vi "Get Active List - By Core Number.vi"(7 "Parameters Array (in)":T1[](array[typedef])) -> (8 "Active Core Numbers":i32[](array[numeric]))   [LabVIEW 2017] (continued)
Number"=0, "Channel Number"=8, "Channel Name"="RDC13_NWS_RX", "Channel Speed"=100, "Label Decimal"=6, "Label Name"="Label_6", "Min Rate (mS)"=40, "Max Rate (mS)"=60, "SDI"=0, "SSM"=0, "Create SDI"=FALSE, "Create SSM"=FALSE, "Create Parity"=FALSE, "Parameter Name"="left_wheel_speed", "Start Bit"=16, "Number of Bits"=13, "Scale"="0.125", "Offset"="0", "Signed"=TRUE, "Unit"="knots", "Encoding"=enum."BNR", "Default Value"="0"}, {"Core Number"=0, "Channel Number"=8, "Channel Name"="RDC13_NWS_RX", "Channel Speed"=100, "Label Decimal"=6, "Label Name"="Label_6", "Min Rate (mS)"=40, "Max Rate (mS)"=60, "SDI"=0, "SSM"=0, "Create SDI"=FALSE, "Create SSM"=FALSE, "Create Parity"=FALSE, "Parameter Name"="sdi", "Start Bit"=8, "Number of Bits"=2, "Scale"="1", "Offset"="0", "Signed"=FALSE, "Unit"="", "Encoding"=enum."BNR", "Default Value"="0"}, {"Core Number"=0, "Channel Number"=8, "Channel Name"="RDC13_NWS_RX", "Channel Speed"=100, "Label Decimal"=7, "Label Name"="Label_7", "Min Rate (mS)"=40, "Max Rate (mS)"=60, "SDI"=0, "SSM"=0, "Create SDI"=FALSE, "Create SSM"=FALSE, "Create Parity"=FALSE, "Parameter Name"="right_wheel_speed", "Start Bit"=16, "Number of Bits"=13, "Scale"="0.125", "Offset"="0", "Signed"=TRUE, "Unit"="knots", "Encoding"=enum."BNR", "Default Value"="0"}, {"Core Number"=0, "Channel Number"=8, "Channel Name"="RDC13_NWS_RX", "Channel Speed"=100, "Label Decimal"=7, "Label Name"="Label_7", "Min Rate (mS)"=40, "Max Rate (mS)"=60, "SDI"=0, "SSM"=0, "Create SDI"=FALSE, "Create SSM"=FALSE, "Create Parity"=FALSE, "Parameter Name"="sdi", "Start Bit"=8, "Number of Bits"=2, "Scale"="1", "Offset"="0", "Signed"=FALSE, "Unit"="", "Encoding"=enum."BNR", "Default Value"="0"}, {"Core Number"=0, "Channel Number"=8, "Channel Name"="RDC13_NWS_RX", "Channel Speed"=100, "Label Decimal"=17, "Label Name"="Label_21", "Min Rate (mS)"=16, "Max Rate (mS)"=24, "SDI"=0, "SSM"=0, "Create SDI"=FALSE, "Create SSM"=FALSE, "Create Parity"=FALSE, "Parameter Name"="gear_down_select", "Start Bit"=26, "Number of Bits"=1, "Scale"="0", "Offset"="0", "Signed"=FALSE, "Unit"="", "Encoding"=enum."Discrete", "Default Value"="0"}, {"Core Number"=0, "Channel Number"=8, "Channel Name"="RDC13_NWS_RX", "Channel Speed"=100, "Label Decimal"=17, "Label Name"="Label_21", "Min Rate (mS)"=16, "Max Rate (mS)"=24, "SDI"=0, "SSM"=0, "Create SDI"=FALSE, "Create SSM"=FALSE, "Create Parity"=FALSE, "Parameter Name"="gear_in_transit_state", "Start Bit"=24, "Number of Bits"=1, "Scale"="0", "Offset"="0", "Signed"=FALSE, "Unit"="", "Encoding"=enum."Discrete", "Default Value"="0"}, {"Core Number"=0, "Channel Number"=8, "Channel Name"="RDC13_NWS_RX", "Channel Speed"=100, "Label Decimal"=17, "Label Name"="Label_21", "Min Rate (mS)"=16, "Max Rate (mS)"=24, "SDI"=0, "SSM"=0, "Create SDI"=FALSE, "Create SSM"=FALSE, "Create Parity"=FALSE, "Parameter Name"="gear_up_select", "Start Bit"=27, "Number of Bits"=1, "Scale"="0", "Offset"="0", "Signed"=FALSE, "Unit"="", "Encoding"=enum."Discrete", "Default Value"="0"}, {"Core Number"=0, "Channel Number"=8, "Channel Name"="RDC13_NWS_RX", "Channel Speed"=100, "Label Decimal"=17, "Label Name"="Label_21", "Min Rate (mS)"=16, "Max Rate (mS)"=24, "SDI"=0, "SSM"=0, "Create SDI"=FALSE, "Create SSM"=FALSE, "Create Parity"=FALSE, "Parameter Name"="lh_mlg_gear_downlock_state", "Start Bit"=18, "Number of Bits"=1, "Scale"="0", "Offset"="0", "Signed"=FALSE, "Unit"="", "Encoding"=enum."Discrete", "Default Value"="0"}, {"Core Number"=0, "Channel Number"=8, "Channel Name"="RDC13_NWS_RX", "Channel Speed"=100, "Label Decimal"=17, "Label Name"="Label_21", "Min Rate (mS)"=16, "Max Rate (mS)"=24, "SDI"=0, "SSM"=0, "Create SDI"=FALSE, "Create SSM"=FALSE, "Create Parity"=FALSE, "Parameter Name"="lh_mlg_gear_downlock_valid", "Start Bit"=19, "Number of Bits"=1, "Scale"="0", "Offset"="0", "Signed"=FALSE, "Unit"="", "Encoding"=enum."Discrete", "Default Value"="0"}, {"Core Number"=0, "Channel Number"=8, "Channel Name"="RDC13_NWS_RX", "Channel Speed"=100, "Label Decimal"=17, "Label Name"="Label_21", "Min Rate (mS)"=16, "Max Rate (mS)"=24, "SDI"=0, "SSM"=0, "Create SDI"=FALSE, "Create SSM"=FALSE, "Create Parity"=FALSE, "Parameter Name"="lh_mlg_gear_uplock_state", "Start Bit"=10, "Number of Bits"=1, "Scale"="0", "Offset"="0", "Signed"=FALSE, "Unit"="", "Encoding"=enum."Discrete", "Default Value"="0"}, {"Core Number"=0, "Channel Number"=8, "Channel Name"="RDC13_NWS_RX", "Channel Speed"=100, "Label Decimal"=17, "Label Name"="Label_21", "Min Rate (mS)"=16, "Max Rate (mS)"=24, "SDI"=0, "SSM"=0, "Create SDI"=FALSE, "Create SSM"=FALSE, "Create Parity"=FALSE, "Parameter Name"="lh_mlg_gear_uplock_valid", "Start Bit"=11, "Number of Bits"=1, "Scale"="0", "Offset"="0", "Signed"=FALSE, "Unit"="", "Encoding"=enum."Discrete", "Default Value"="0"}, {"Core Number"=0, "Channel Number"=8, "Channel Name"="RDC13_NWS_RX", "Channel Speed"=100, "Label Decimal"=17, "Label Name"="Label_21", "Min Rate (mS)"=16, "Max Rate (mS)"=24, "SDI"=0, "SSM"=0, "Create SDI"=FALSE, "Create SSM"=FALSE, "Create Parity"=FALSE, "Parameter Name"="maint_mode_mlg_extend_selected", "Start Bit"=28, "Number of Bits"=1, "Scale"="0", "Offset"="0", "Signed"=FALSE, "Unit"="", "Encoding"=enum."Discrete", "Default Value"="0"}, {"Core Number"=0, "Channel Number"=8, "Channel Name"="RDC13_NWS_RX", "Channel Speed"=100, "Label Decimal"=17, "Label Name"="Label_21", "Min Rate (mS)"=16, "Max Rate (mS)"=24, "SDI"=0, "SSM"=0, "Create SDI"=FALSE, "Create SSM"=FALSE, "Create Parity"=FALSE, "Parameter Name"="maint_mode_mlg_retract_selected", "Start Bit"=17, "Number of Bits"=1, "Scale"="0", "Offset"="0", "Signed"=FALSE, "Unit"="", "Encoding"=enum."Discrete", "Default Value"="0"}, {"Core Number"=0, "Channel Number"=8, "Channel Name"="RDC13_NWS_RX", "Channel Speed"=100, "Label Decimal"=17, "Label Name"="Label_21", "Min Rate (mS)"=16, "Max Rate (mS)"=24, "SDI"=0, "SSM"=0, "Create SDI"=FALSE, "Create SSM"=FALSE, "Create Parity"=FALSE, "Parameter Name"="nlg_gear_downlock_state", "Start Bit"=22, "Number of Bits"=1, "Scale"="0", "Offset"="0", "Signed"=FALSE, "Unit"="", "Encoding"=enum."Discrete", "Default Value"="0"}, {"Core Number"=0, "Channel Number"=8, "Channel Name"="RDC13_NWS_RX", "Channel Speed"=100, "Label Decimal"=17, "Label Name"="Label_21", "Min Rate (mS)"=16, "Max Rate (mS)"=24, "SDI"=0, "SSM"=0, "Create SDI"=FALSE, "Create SSM"=FALSE, "Create Parity"=FALSE, "Parameter Name"="nlg_gear_downlock_valid", "Start Bit"=23, "Number of Bits"=1, "Scale"="0", "Offset"="0", "Signed"=FALSE, "Unit"="", "Encoding"=enum."Discrete", "Default Value"="0"}, {"Core Number"=0, "Channel Number"=8, "Channel Name"="RDC13_NWS_RX", "Channel Speed"=100, "Label Decimal"=17, "Label Name"="Label_21", "Min Rate (mS)"=16, "Max Rate (mS)"=24, "SDI"=0, "SSM"=0, "Create SDI"=FALSE, "Create SSM"=FALSE, "Create Parity"=FALSE, "Parameter Name"="nlg_gear_uplock_state", "Start Bit"=14, "Number of Bits"=1, "Scale"="0", "Offset"="0", "Signed"=FALSE, "Unit"="", "Encoding"=enum."Discrete", "Default Value"="0"}, {"Core Number"=0, "Channel Number"=8, "Channel Name"="RDC13_NWS_RX", "Channel Speed"=100, "Label Decimal"=17, "Label Name"="Label_21", "Min Rate (mS)"=16, "Max Rate (mS)"=24, "SDI"=0, "SSM"=0, "Create SDI"=FALSE, "Create SSM"=FALSE, "Create Parity"=FALSE, "Parameter Name"="nlg_gear_uplock_valid", "Start Bit"=15, "Number of Bits"=1, "Scale"="0", "Offset"="0", "Signed"=FALSE, "Unit"="", "Encoding"=enum."Discrete", "Default Value"="0"}, {"Core Number"=0, "Channel Number"=8, "Channel Name"="RDC13_NWS_RX", "Channel Speed"=100, "Label Decimal"=17, "Label Name"="Label_21", "Min Rate (mS)"=16, "Max Rate (mS)"=24, "SDI"=0, "SSM"=0, "Create SDI"=FALSE, "Create SSM"=FALSE, "Create Parity"=FALSE, "Parameter Name"="nose_wheel_centered", "Start Bit"=16, "Number of Bits"=1, "Scale"="0", "Offset"="0", "Signed"=FALSE, "Unit"="", "Encoding"=enum."Discrete", "Default Value"="0"}, {"Core Number"=0, "Channel Number"=8, "Channel Name"="RDC13_NWS_RX", "Channel Speed"=100, "Label Decimal"=17, "Label Name"="Label_21", "Min Rate (mS)"=16, "Max Rate (mS)"=24, "SDI"=0, "SSM"=0, "Create SDI"=FALSE, "Create SSM"=FALSE, "Create Parity"=FALSE, "Parameter Name"="rh_mlg_gear_downlock_state", "Start Bit"=20, "Number of Bits"=1, "Scale"="0", "Offset"="0", "Signed"=FALSE, "Unit"="", "Encoding"=enum."Discrete", "Default Value"="0"}, {"Core Number"=0, "Channel Number"=8, "Channel Name"="RDC13_NWS_RX", "Channel Speed"=100, "Label Decimal"=17, "Label Name"="Label_21", "Min Rate (mS)"=16, "Max Rate (mS)"=24, "SDI"=0, "SSM"=0, "Create SDI"=FALSE, "Create SSM"=FALSE, "Create Parity"=FALSE, "Parameter Name"="rh_mlg_gear_downlock_valid", "Start Bit"=21, "Number of Bits"=1, "Scale"="0", "Offset"="0", "Signed"=FALSE, "Unit"="", "Encoding"=enum."Discrete", "Default Value"="0"}, {"Core Number"=0, "Channel Number"=8, "Channel Name"="RDC13_NWS_RX", "Channel Speed"=100, "Label Decimal"=17, "Label Name"="Label_21", "Min Rate (mS)"=16, "Max Rate (mS)"=24, "SDI"=0, "SSM"=0, "Create SDI"=FALSE, "Create SSM"=FALSE, "Create Parity"=FALSE, "Parameter Name"="rh_mlg_gear_uplock_state", "Start Bit"=12, "Number of Bits"=1, "Scale"="0", "Offset"="0", "Signed"=FALSE, "Unit"="", "Encoding"=enum."Discrete", "Default Value"="0"}, {"Core Number"=0, "Channel Number"=8, "Channel Name"="RDC13_NWS_RX", "Channel Speed"=100, "Label Decimal"=17, "Label Name"="Label_21", "Min Rate (mS)"=16, "Max Rate (mS)"=24, "SDI"=0, "SSM"=0, "Create SDI"=FALSE, "Create SSM"=FALSE, "Create Parity"=FALSE, "Parameter Name"="rh_mlg_gear_uplock_valid", "Start Bit"=13, "Number of Bits"=1, "Scale"="0", "Offset"="0", "Signed"=FALSE, "Unit"="", "Encoding"=enum."Discrete", "Default Value"="0"}, {"Core Number"=0, "Channel Number"=8, "Channel Name"="RDC13_NWS_RX", "Channel Speed"=100, "Label Decimal"=17, "Label Name"="Label_21", "Min Rate (mS)"=16, "Max Rate (mS)"=24, "SDI"=0, "SSM"=0, "Create SDI"=FALSE, "Create SSM"=FALSE, "Create Parity"=FALSE, "Parameter Name"="sdi", "Start Bit"=8, "Number of Bits"=2, "Scale"="1", "Offset"="0", "Signed"=FALSE, "Unit"="", "Encoding"=enum."BNR", "Default Value"="0"}, {"Core Number"=0, "Channel Number"=8, "Channel Name"="RDC13_NWS_RX", "Channel Speed"=100, "Label Decimal"=18, "Label Name"="Label_22", "Min Rate (mS)"=16, "Max Rate (mS)"=24, "SDI"=0, "SSM"=0, "Create SDI"=FALSE, "Create SSM"=FALSE, "Create Parity"=FALSE, "Parameter Name"="all_gear_not_uplocked_state", "Start Bit"=22, "Number of Bits"=1, "Scale"="0", "Offset"="0", "Signed"=FALSE, "Unit"="", "Encoding"=enum."Discrete", "Default Value"="0"}, {"Core Number"=0, "Channel Number"=8, "Channel Name"="RDC13_NWS_RX", "Channel Speed"=100, "Label Decimal"=18, "Label Name"="Label_22", "Min Rate (mS)"=16, "Max Rate (mS)"=24, "SDI"=0, "SSM"=0, "Create SDI"=FALSE, "Create SSM"=FALSE, "Create Parity"=FALSE, "Parameter Name"="all_gear_not_uplocked_valid", "Start Bit"=23, "Number of Bits"=1, "Scale"="0", "Offset"="0", "Signed"=FALSE, "Unit"="", "Encoding"=enum."Discrete", "Default Value"="0"}, {"Core Number"=0, "Channel Number"=8, "Channel Name"="RDC13_NWS_RX", "Channel Speed"=100, "Label Decimal"=18, "Label Name"="Label_22", "Min Rate (mS)"=16, "Max Rate (mS)"=24, "SDI"=0, "SSM"=0, "Create SDI"=FALSE, "Create SSM"=FALSE, "Create Parity"=FALSE, "Parameter Name"="comb_l_or_r_main_gear_downlocked_state", "Start Bit"=16, "Number of Bits"=1, "Scale"="0", "Offset"="0", "Signed"=FALSE, "Unit"="", "Encoding"=enum."Discrete", "Default Value"="0"}, {"Core Number"=0, "Channel Number"=8, "Channel Name"="RDC13_NWS_RX", "Channel Speed"=100, "Label Decimal"=18, "Label Name"="Label_22", "Min Rate (mS)"=16, "Max Rate (mS)"=24, "SDI"=0, "SSM"=0, "Create SDI"=FALSE, "Create SSM"=FALSE, "Create Parity"=FALSE, "Parameter Name"="comb_l_or_r_main_gear_downlocked_valid", "Start Bit"=17, "Number of Bits"=1, "Scale"="0", "Offset"="0", "Signed"=FALSE, "Unit"="", "Encoding"=enum."Discrete", "Default Value"="0"}, {"Core Number"=0, "Channel Number"=8, "Channel Name"="RDC13_NWS_RX", "Channel Speed"=100, "Label Decimal"=18, "Label Name"="Label_22", "Min Rate (mS)"=16, "Max Rate (mS)"=24, "SDI"=0, "SSM"=0, "Create SDI"=FALSE, "Create SSM"=FALSE, "Create Parity"=FALSE, "Parameter Name"="comb_lh_or_rh_mlg_not_wow", "Start Bit"=20, "Number of Bits"=1, "Scale"="0", "Offset"="0", "Signed"=FALSE, "Unit"="", "Encoding"=enum."Discrete", "Default Value"="0"}, {"Core Number"=0, "Channel Number"=8, "Channel Name"="RDC13_NWS_RX", "Channel Speed"=100, "Label Decimal"=18, "Label Name"="Label_22", "Min Rate (mS)"=16, "Max Rate (mS)"=24, "SDI"=0, "SSM"=0, "Create SDI"=FALSE, "Create SSM"=FALSE, "Create Parity"=FALSE, "Parameter Name"="comb_lh_or_rh_mlg_wow", "Start Bit"=18, "Number of Bits"=1, "Scale"="0", "Offset"="0", "Signed"=FALSE, "Unit"="", "Encoding"=enum."Discrete", "Default Value"="0"}, {"Core Number"=0, "Channel Number"=8, "Channel Name"="RDC13_NWS_RX", "Channel Speed"=100, "Label Decimal"=18, "Label Name"="Label_22", "Min Rate (mS)"=16, "Max Rate (mS)"=24, "SDI"=0, "SSM"=0, "Create SDI"=FALSE, "Create SSM"=FALSE, "Create Parity"=FALSE, "Parameter Name"="lh_mlg_wow_state", "Start Bit"=10, "Number of Bits"=1, "Scale"="0", "Offset"="0", "Signed"=FALSE, "Unit"="", "Encoding"=enum."Discrete", "Default Value"="0"}, {"Core Number"=0, "Channel Number"=8, "Channel Name"="RDC13_NWS_RX", "Channel Speed"=100, "Label Decimal"=18, "Label Name"="Label_22", "Min Rate (mS)"=16, "Max Rate (mS)"=24, "SDI"=0, "SSM"=0, "Create SDI"=FALSE, "Create SSM"=FALSE, "Create Parity"=FALSE, "Parameter Name"="lh_mlg_wow_valid", "Start Bit"=11, "Number of Bits"=1, "Scale"="0", "Offset"="0", "Signed"=FALSE, "Unit"="", "Encoding"=enum."Discrete", "Default Value"="0"}, {"Core Number"=0, "Channel Number"=8, "Channel Name"="RDC13_NWS_RX", "Channel Speed"=100, "Label Decimal"=18, "Label Name"="Label_22", "Min Rate (mS)"=16, "Max Rate (mS)"=24, "SDI"=0, "SSM"=0, "Create SDI"=FALSE, "Create SSM"=FALSE, "Create Parity"=FALSE, "Parameter Name"="lh_or_rh_mlg_not_wow_valid", "Start Bit"=21, "Number of Bits"=1, "Scale"="0", "Offset"="0", "Signed"=FALSE, "Unit"="", "Encoding"=enum."Discrete", "Default Value"="0"}, {"Core Number"=0, "Channel Number"=8, "Channel Name"="RDC13_NWS_RX", "Channel Speed"=100, "Label Decimal"=18, "Label Name"="Label_22", "Min Rate (mS)"=16, "Max Rate (mS)"=24, "SDI"=0, "SSM"=0, "Create SDI"=FALSE, "Create SSM"=FALSE, "Create Parity"=FALSE, "Parameter Name"="lh_or_rh_mlg_wow_valid", "Start Bit"=19, "Number of Bits"=1, "Scale"="0", "Offset"="0", "Signed"=FALSE, "Unit"="", "Encoding"=enum."Discrete", "Default Value"="0"}, {"Core Number"=0, "Channel Number"=8, "Channel Name"="RDC13_NWS_RX", "Channel Speed"=100, "Label Decimal"=18, "Label Name"="Label_22", "Min Rate (mS)"=16, "Max Rate (mS)"=24, "SDI"=0, "SSM"=0, "Create SDI"=FALSE, "Create SSM"=FALSE, "Create Parity"=FALSE, "Parameter Name"="maint_mode_nlg_extend_selected", "Start Bit"=25, "Number of Bits"=1, "Scale"="0", "Offset"="0", "Signed"=FALSE, "Unit"="", "Encoding"=enum."Discrete", "Default Value"="0"}, {"Core Number"=0, "Channel Number"=8, "Channel Name"="RDC13_NWS_RX", "Channel Speed"=100, "Label Decimal"=18, "Label Name"="Label_22", "Min Rate (mS)"=16, "Max Rate (mS)"=24, "SDI"=0, "SSM"=0, "Create SDI"=FALSE, "Create SSM"=FALSE, "Create Parity"=FALSE, "Parameter Name"="maint_mode_nlg_retract_selected", "Start Bit"=24, "Number of Bits"=1, "Scale"="0", "Offset"="0", "Signed"=FALSE, "Unit"="", "Encoding"=enum."Discrete", "Default Value"="0"}, {"Core Number"=0, "Channel Number"=8, "Channel Name"="RDC13_NWS_RX", "Channel Speed"=100, "Label Decimal"=18, "Label Name"="Label_22", "Min Rate (mS)"=16, "Max Rate (mS)"=24, "SDI"=0, "SSM"=0, "Create SDI"=FALSE, "Create SSM"=FALSE, "Create Parity"=FALSE, "Parameter Name"="maint_mode_selected", "Start Bit"=28, "Number of Bits"=1, "Scale"="0", "Offset"="0", "Signed"=FALSE, "Unit"="", "Encoding"=enum."Discrete", "Default Value"="0"}, {"Core Number"=0, "Channel Number"=8, "Channel Name"="RDC13_NWS_RX", "Channel Speed"=100, "Label Decimal"=18, "Label Name"="Label_22", "Min Rate (mS)"=16, "Max Rate (mS)"=24, "SDI"=0, "SSM"=0, "Create SDI"=FALSE, "Create SSM"=FALSE, "Create Parity"=FALSE, "Parameter Name"="maint_mode_wow_in_air_selected", "Start Bit"=27, "Number of Bits"=1, "Scale"="0", "Offset"="0", "Signed"=FALSE, "Unit"="", "Encoding"=enum."Discrete", "Default Value"="0"}, {"Core Number"=0, "Channel Number"=8, "Channel Name"="RDC13_NWS_RX", "Channel Speed"=100, "Label Decimal"=18, "Label Name"="Label_22", "Min Rate (mS)"=16, "Max Rate (mS)"=24, "SDI"=0, "SSM"=0, "Create SDI"=FALSE, "Create SSM"=FALSE, "Create Parity"=FALSE, "Parameter Name"="maint_mode_wow_on_ground_selected", "Start Bit"=26, "Number of Bits"=1, "Scale"="0", "Offset"="0", "Signed"=FALSE, "Unit"="", "Encoding"=enum."Discrete", "Default Value"="0"}, {"Core Number"=0, "Channel Number"=8, "Channel Name"="RDC13_NWS_RX", "Channel Speed"=100, "Label Decimal"=18, "Label Name"="Label_22", "Min Rate (mS)"=16, "Max Rate (mS)"=24, "SDI"=0, "SSM"=0, "Create SDI"=FALSE, "Create SSM"=FALSE, "Create Parity"=FALSE, "Parameter Name"="nlg_wow_state", "Start Bit"=14, "Number of Bits"=1, "Scale"="0", "Offset"="0", "Signed"=FALSE, "Unit"="", "Encoding"=enum."Discrete", "Default Value"="0"}, {"Core Number"=0, "Channel Number"=8, "Channel Name"="RDC13_NWS_RX", "Channel Speed"=100, "Label Decimal"=18, "Label Name"="Label_22", "Min Rate (mS)"=16, "Max Rate (mS)"=24, "SDI"=0, "SSM"=0, "Create SDI"=FALSE, "Create SSM"=FALSE, "Create Parity"=FALSE, "Parameter Name"="nlg_wow_valid", "Start Bit"=15, "Number of Bits"=1, "Scale"="0", "Offset"="0", "Signed"=FALSE, "Unit"="", "Encoding"=enum."Discrete", "Default Value"="0"}, {"Core Number"=0, "Channel Number"=8, "Channel Name"="RDC13_NWS_RX", "Channel Speed"=100, "Label Decimal"=18, "Label Name"="Label_22", "Min Rate (mS)"=16, "Max Rate (mS)"=24, "SDI"=0, "SSM"=0, "Create SDI"=FALSE, "Create SSM"=FALSE, "Create Parity"=FALSE, "Parameter Name"="rh_mlg_wow_state", "Start Bit"=12, "Number of Bits"=1, "Scale"="0", "Offset"="0", "Signed"=FALSE, "Unit"="", "Encoding"=enum."Discrete", "Default Value"="0"}, {"Core Number"=0, "Channel Number"=8, "Channel Name"="RDC13_NWS_RX", "Channel Speed"=100, "Label Decimal"=18, "Label Name"="Label_22", "Min Rate (mS)"=16, "Max Rate (mS)"=24, "SDI"=0, "SSM"=0, "Create SDI"=FALSE, "Create SSM"=FALSE, "Create Parity"=FALSE, "Parameter Name"="rh_mlg_wow_valid", "Start Bit"=13, "Number of Bits"=1, "Scale"="0", "Offset"="0", "Signed"=FALSE, "Unit"="", "Encoding"=enum."Discrete", "Default Value"="0"}, {"Core Number"=0, "Channel Number"=8, "Channel Name"="RDC13_NWS_RX", "Channel Speed"=100, "Label Decimal"=18, "Label Name"="Label_22", "Min Rate (mS)"=16, "Max Rate (mS)"=24, "SDI"=0, "SSM"=0, "Create SDI"=FALSE, "Create SSM"=FALSE, "Create Parity"=FALSE, "Parameter Name"="sdi", "Start Bit"=8, "Number of Bits"=2, "Scale"="1", "Offset"="0", "Signed"=FALSE, "Unit"="", "Encoding"=enum."BNR", "Default Value"="0"}, {"Core Number"=0, "Channel Number"=8, "Channel Name"="RDC13_NWS_RX", "Channel Speed"=100, "Label Decimal"=85, "Label Name"="Label_125", "Min Rate (mS)"=96, "Max Rate (mS)"=144, "SDI"=0, "SSM"=0, "Create SDI"=FALSE, "Create SSM"=FALSE, "Create Parity"=FALSE, "Parameter Name"="ac_time_hours_ones", "Start Bit"=22, "Number of Bits"=4, "Scale"="1", "Offset"="0", "Signed"=FALSE, "Unit"="hours", "Encoding"=enum."BNR", "Default Value"="0"}, {"Core Number"=0, "Channel Number"=8, "Channel Name"="RDC13_NWS_RX", "Channel Speed"=100, "Label Decimal"=85, "Label Name"="Label_125", "Min Rate (mS)"=96, "Max Rate (mS)"=144, "SDI"=0, "SSM"=0, "Create SDI"=FALSE, "Create SSM"=FALSE, "Create Parity"=FALSE, "Parameter Name"="ac_time_hours_tens", "Start Bit"=26, "Number of Bits"=2, "Scale"="10", "Offset"="0", "Signed"=FALSE, "Unit"="hours", "Encoding"=enum."BNR", "Default Value"="0"}, {"Core Number"=0, "Channel Number"=8, "Channel Name"="RDC13_NWS_RX", "Channel Speed"=100, "Label Decimal"=85, "Label Name"="Label_125", "Min Rate (mS)"=96, "Max Rate (mS)"=144, "SDI"=0, "SSM"=0, "Create SDI"=FALSE, "Create SSM"=FALSE, "Create Parity"=FALSE, "Parameter Name"="ac_time_minutes_ones", "Start Bit"=14, "Number of Bits"=4, "Scale"="1", "Offset"="0", "Signed"=FALSE, "Unit"="minutes", "Encoding"=enum."BNR", "Default Value"="0"}, {"Core Number"=0, "Channel Number"=8, "Channel Name"="RDC13_NWS_RX", "Channel Speed"=100, "Label Decimal"=85, "Label Name"="Label_125", "Min Rate (mS)"=96, "Max Rate (mS)"=144, "SDI"=0, "SSM"=0, "Create SDI"=FALSE, "Create SSM"=FALSE, "Create Parity"=FALSE, "Parameter Name"="ac_time_minutes_tens", "Start Bit"=18, "Number of Bits"=4, "Scale"="10", "Offset"="0", "Signed"=FALSE, "Unit"="minutes", "Encoding"=enum."BNR", "Default Value"="0"}, {"Core Number"=0, "Channel Number"=8, "Channel Name"="RDC13_NWS_RX", "Channel Speed"=100, "Label Decimal"=85, "Label Name"="Label_125", "Min Rate (mS)"=96, "Max Rate (mS)"=144, "SDI"=0, "SSM"=0, "Create SDI"=FALSE, "Create SSM"=FALSE, "Create Parity"=FALSE, "Parameter Name"="ac_time_minutes_tenths", "Start Bit"=10, "Number of Bits"=4, "Scale"="0.1", "Offset"="0", "Signed"=FALSE, "Unit"="minutes", "Encoding"=enum."BNR", "Default Value"="0"}, {"Core Number"=0, "Channel Number"=8, "Channel Name"="RDC13_NWS_RX", "Channel Speed"=100, "Label Decimal"=85, "Label Name"="Label_125", "Min Rate (mS)"=96, "Max Rate (mS)"=144, "SDI"=0, "SSM"=0, "Create SDI"=FALSE, "Create SSM"=FALSE, "Create Parity"=FALSE, "Parameter Name"="sdi", "Start Bit"=8, "Number of Bits"=2, "Scale"="1", "Offset"="0", "Signed"=FALSE, "Unit"="", "Encoding"=enum."BNR", "Default Value"="0"}, {"Core Number"=0, "Channel Number"=8, "Channel Name"="RDC13_NWS_RX", "Channel Speed"=100, "Label Decimal"=86, "Label Name"="Label_126", "Min Rate (mS)"=800, "Max Rate (mS)"=1200, "SDI"=0, "SSM"=0, "Create SDI"=FALSE, "Create SSM"=FALSE, "Create Parity"=FALSE, "Parameter Name"="ac_flight_phase", "Start Bit"=19, "Number of Bits"=4, "Scale"="1", "Offset"="0", "Signed"=TRUE, "Unit"="", "Encoding"=enum."BNR", "Default Value"="0"}, {"Core Number"=0, "Channel Number"=8, "Channel Name"="RDC13_NWS_RX", "Channel Speed"=100, "Label Decimal"=86, "Label Name"="Label_126", "Min Rate (mS)"=800, "Max Rate (mS)"=1200, "SDI"=0, "SSM"=0, "Create SDI"=FALSE, "Create SSM"=FALSE, "Create Parity"=FALSE, "Parameter Name"="sdi", "Start Bit"=8, "Number of Bits"=2, "Scale"="1", "Offset"="0", "Signed"=FALSE, "Unit"="", "Encoding"=enum."BNR", "Default Value"="0"}, {"Core Number"=0, "Channel Number"=8, "Channel Name"="RDC13_NWS_RX", "Channel Speed"=100, "Label Decimal"=125, "Label Name"="Label_175", "Min Rate (mS)"=32, "Max Rate (mS)"=48, "SDI"=0, "SSM"=0, "Create SDI"=FALSE, "Create SSM"=FALSE, "Create Parity"=FALSE, "Parameter Name"="hybrid_ground_speed", "Start Bit"=10, "Number of Bits"=19, "Scale"="0.01565", "Offset"="0", "Signed"=TRUE, "Unit"="knots", "Encoding"=enum."BNR", "Default Value"="0"}, {"Core Number"=0, "Channel Number"=8, "Channel Name"="RDC13_NWS_RX", "Channel Speed"=100, "Label Decimal"=125, "Label Name"="Label_175", "Min Rate (mS)"=32, "Max Rate (mS)"=48, "SDI"=0, "SSM"=0, "Create SDI"=FALSE, "Create SSM"=FALSE, "Create Parity"=FALSE, "Parameter Name"="sdi", "Start Bit"=8, "Number of Bits"=2, "Scale"="1", "Offset"="0", "Signed"=FALSE, "Unit"="", "Encoding"=enum."BNR", "Default Value"="0"}, {"Core Number"=0, "Channel Number"=8, "Channel Name"="RDC13_NWS_RX", "Channel Speed"=100, "Label Decimal"=136, "Label Name"="Label_210", "Min Rate (mS)"=512, "Max Rate (mS)"=768, "SDI"=0, "SSM"=0, "Create SDI"=FALSE, "Create SSM"=FALSE, "Create Parity"=FALSE, "Parameter Name"="left_hydraulic_pressure", "Start Bit"=15, "Number of Bits"=13, "Scale"="0.5", "Offset"="0", "Signed"=TRUE, "Unit"="psi", "Encoding"=enum."BNR", "Default Value"="0"}, {"Core Number"=0, "Channel Number"=8, "Channel Name"="RDC13_NWS_RX", "Channel Speed"=100, "Label Decimal"=136, "Label Name"="Label_210", "Min Rate (mS)"=512, "Max Rate (mS)"=768, "SDI"=0, "SSM"=0, "Create SDI"=FALSE, "Create SSM"=FALSE, "Create Parity"=FALSE, "Parameter Name"="sdi", "Start Bit"=8, "Number of Bits"=2, "Scale"="1", "Offset"="0", "Signed"=FALSE, "Unit"="", "Encoding"=enum."BNR", "Default Value"="0"}, {"Core Number"=0, "Channel Number"=8, "Channel Name"="RDC13_NWS_RX", "Channel Speed"=100, "Label Decimal"=138, "Label Name"="Label_212", "Min Rate (mS)"=512, "Max Rate (mS)"=768, "SDI"=0, "SSM"=0, "Create SDI"=FALSE, "Create SSM"=FALSE, "Create Parity"=FALSE, "Parameter Name"="auxiliary_hudraulic_pressure", "Start Bit"=15, "Number of Bits"=13, "Scale"="0.5", "Offset"="0", "Signed"=TRUE, "Unit"="psi", "Encoding"=enum."BNR", "Default Value"="0"}, {"Core Number"=0, "Channel Number"=8, "Channel Name"="RDC13_NWS_RX", "Channel Speed"=100, "Label Decimal"=138, "Label Name"="Label_212", "Min Rate (mS)"=512, "Max Rate (mS)"=768, "SDI"=0, "SSM"=0, "Create SDI"=FALSE, "Create SSM"=FALSE, "Create Parity"=FALSE, "Parameter Name"="sdi", "Start Bit"=8, "Number of Bits"=2, "Scale"="1", "Offset"="0", "Signed"=FALSE, "Unit"="", "Encoding"=enum."BNR", "Default Value"="0"}, {"Core Number"=0, "Channel Number"=8, "Channel Name"="RDC13_NWS_RX", "Channel Speed"=100, "Label Decimal"=139, "Label Name"="Label_213", "Min Rate (mS)"=800, "Max Rate (mS)"=1200, "SDI"=0, "SSM"=0, "Create SDI"=FALSE, "Create SSM"=FALSE, "Create Parity"=FALSE, "Parameter Name"="ptu_pressure", "Start Bit"=15, "Number of Bits"=13, "Scale"="0.5", "Offset"="0", "Signed"=TRUE, "Unit"="psi", "Encoding"=enum."BNR", "Default Value"="0"}, {"Core Number"=0, "Channel Number"=8, "Channel Name"="RDC13_NWS_RX", "Channel Speed"=100, "Label Decimal"=139, "Label Name"="Label_213", "Min Rate (mS)"=800, "Max Rate (mS)"=1200, "SDI"=0, "SSM"=0, "Create SDI"=FALSE, "Create SSM"=FALSE, "Create Parity"=FALSE, "Parameter Name"="sdi", "Start Bit"=8, "Number of Bits"=2, "Scale"="1", "Offset"="0", "Signed"=FALSE, "Unit"="", "Encoding"=enum."BNR", "Default Value"="0"}, {"Core Number"=0, "Channel Number"=8, "Channel Name"="RDC13_NWS_RX", "Channel Speed"=100, "Label Decimal"=150, "Label Name"="Label_226", "Min Rate (mS)"=800, "Max Rate (mS)"=1200, "SDI"=0, "SSM"=0, "Create SDI"=FALSE, "Create SSM"=FALSE, "Create Parity"=FALSE, "Parameter Name"="ac_ser_num_hundreds", "Start Bit"=14, "Number of Bits"=4, "Scale"="100", "Offset"="0", "Signed"=TRUE, "Unit"="", "Encoding"=enum."BNR", "Default Value"="0"}, {"Core Number"=0, "Channel Number"=8, "Channel Name"="RDC13_NWS_RX", "Channel Speed"=100, "Label Decimal"=150, "Label Name"="Label_226", "Min Rate (mS)"=800, "Max Rate (mS)"=1200, "SDI"=0, "SSM"=0, "Create SDI"=FALSE, "Create SSM"=FALSE, "Create Parity"=FALSE, "Parameter Name"="ac_ser_num_ones", "Start Bit"=22, "Number of Bits"=4, "Scale"="1", "Offset"="0", "Signed"=TRUE, "Unit"="", "Encoding"=enum."BNR", "Default Value"="0"}, {"Core Number"=0, "Channel Number"=8, "Channel Name"="RDC13_NWS_RX", "Channel Speed"=100, "Label Decimal"=150, "Label Name"="Label_226", "Min Rate (mS)"=800, "Max Rate (mS)"=1200, "SDI"=0, "SSM"=0, "Create SDI"=FALSE, "Create SSM"=FALSE, "Create Parity"=FALSE, "Parameter Name"="ac_ser_num_tens", "Start Bit"=18, "Number of Bits"=4, "Scale"="10", "Offset"="0", "Signed"=TRUE, "Unit"="", "Encoding"=enum."BNR", "Default Value"="0"}, {"Core Number"=0, "Channel Number"=8, "Channel Name"="RDC13_NWS_RX", "Channel Speed"=100, "Label Decimal"=150, "Label Name"="Label_226", "Min Rate (mS)"=800, "Max Rate (mS)"=1200, "SDI"=0, "SSM"=0, "Create SDI"=FALSE, "Create SSM"=FALSE, "Create Parity"=FALSE, "Parameter Name"="ac_ser_num_thousands", "Start Bit"=10, "Number of Bits"=4, "Scale"="1000", "Offset"="0", "Signed"=TRUE, "Unit"="", "Encoding"=enum."BNR", "Default Value"="0"}, {"Core Number"=0, "Channel Number"=8, "Channel Name"="RDC13_NWS_RX", "Channel Speed"=100, "Label Decimal"=150, "Label Name"="Label_226", "Min Rate (mS)"=800, "Max Rate (mS)"=1200, "SDI"=0, "SSM"=0, "Create SDI"=FALSE, "Create SSM"=FALSE, "Create Parity"=FALSE, "Parameter Name"="sdi", "Start Bit"=8, "Number of Bits"=2, "Scale"="1", "Offset"="0", "Signed"=FALSE, "Unit"="", "Encoding"=enum."BNR", "Default Value"="0"}, {"Core Number"=0, "Channel Number"=8, "Channel Name"="RDC13_NWS_RX", "Channel Speed"=100, "Label Decimal"=151, "Label Name"="Label_227", "Min Rate (mS)"=800, "Max Rate (mS)"=1200, "SDI"=0, "SSM"=0, "Create SDI"=FALSE, "Create SSM"=FALSE, "Create Parity"=FALSE, "Parameter Name"="cmc_command", "Start Bit"=18, "Number of Bits"=8, "Scale"="1", "Offset"="0", "Signed"=TRUE, "Unit"="", "Encoding"=enum."BNR", "Default Value"="0"}, {"Core Number"=0, "Channel Number"=8, "Channel Name"="RDC13_NWS_RX", "Channel Speed"=100, "Label Decimal"=151, "Label Name"="Label_227", "Min Rate (mS)"=800, "Max Rate (mS)"=1200, "SDI"=0, "SSM"=0, "Create SDI"=FALSE, "Create SSM"=FALSE, "Create Parity"=FALSE, "Parameter Name"="cmc_command_active", "Start Bit"=28, "Number of Bits"=1, "Scale"="1", "Offset"="0", "Signed"=FALSE, "Unit"="", "Encoding"=enum."Discrete", "Default Value"="0"}, {"Core Number"=0, "Channel Number"=8, "Channel Name"="RDC13_NWS_RX", "Channel Speed"=100, "Label Decimal"=151, "Label Name"="Label_227", "Min Rate (mS)"=800, "Max Rate (mS)"=1200, "SDI"=0, "SSM"=0, "Create SDI"=FALSE, "Create SSM"=FALSE, "Create Parity"=FALSE, "Parameter Name"="cmc_command_equipment_id", "Start Bit"=10, "Number of Bits"=8, "Scale"="1", "Offset"="0", "Signed"=TRUE, "Unit"="", "Encoding"=enum."BNR", "Default Value"="0"}, {"Core Number"=0, "Channel Number"=8, "Channel Name"="RDC13_NWS_RX", "Channel Speed"=100, "Label Decimal"=151, "Label Name"="Label_227", "Min Rate (mS)"=800, "Max Rate (mS)"=1200, "SDI"=0, "SSM"=0, "Create SDI"=FALSE, "Create SSM"=FALSE, "Create Parity"=FALSE, "Parameter Name"="cmc_command_reserved", "Start Bit"=26, "Number of Bits"=2, "Scale"="1", "Offset"="0", "Signed"=TRUE, "Unit"="", "Encoding"=enum."BNR", "Default Value"="0"}, {"Core Number"=0, "Channel Number"=8, "Channel Name"="RDC13_NWS_RX", "Channel Speed"=100, "Label Decimal"=151, "Label Name"="Label_227", "Min Rate (mS)"=800, "Max Rate (mS)"=1200, "SDI"=0, "SSM"=0, "Create SDI"=FALSE, "Create SSM"=FALSE, "Create Parity"=FALSE, "Parameter Name"="sdi", "Start Bit"=8, "Number of Bits"=2, "Scale"="1", "Offset"="0", "Signed"=FALSE, "Unit"="", "Encoding"=enum."BNR", "Default Value"="0"}, {"Core Number"=0, "Channel Number"=8, "Channel Name"="RDC13_NWS_RX", "Channel Speed"=100, "Label Decimal"=176, "Label Name"="Label_260", "Min Rate (mS)"=96, "Max Rate (mS)"=144, "SDI"=0, "SSM"=0, "Create SDI"=FALSE, "Create SSM"=FALSE, "Create Parity"=FALSE, "Parameter Name"="ac_date_day_ones", "Start Bit"=23, "Number of Bits"=4, "Scale"="1", "Offset"="0", "Signed"=FALSE, "Unit"="", "Encoding"=enum."BNR", "Default Value"="0"}, {"Core Number"=0, "Channel Number"=8, "Channel Name"="RDC13_NWS_RX", "Channel Speed"=100, "Label Decimal"=176, "Label Name"="Label_260", "Min Rate (mS)"=96, "Max Rate (mS)"=144, "SDI"=0, "SSM"=0, "Create SDI"=FALSE, "Create SSM"=FALSE, "Create Parity"=FALSE, "Parameter Name"="ac_date_day_tens", "Start Bit"=27, "Number of Bits"=2, "Scale"="1", "Offset"="0", "Signed"=FALSE, "Unit"="", "Encoding"=enum."BNR", "Default Value"="0"}, {"Core Number"=0, "Channel Number"=8, "Channel Name"="RDC13_NWS_RX", "Channel Speed"=100, "Label Decimal"=176, "Label Name"="Label_260", "Min Rate (mS)"=96, "Max Rate (mS)"=144, "SDI"=0, "SSM"=0, "Create SDI"=FALSE, "Create SSM"=FALSE, "Create Parity"=FALSE, "Parameter Name"="ac_date_month_ones", "Start Bit"=18, "Number of Bits"=4, "Scale"="1", "Offset"="0", "Signed"=FALSE, "Unit"="", "Encoding"=enum."BNR", "Default Value"="0"}, {"Core Number"=0, "Channel Number"=8, "Channel Name"="RDC13_NWS_RX", "Channel Speed"=100, "Label Decimal"=176, "Label Name"="Label_260", "Min Rate (mS)"=96, "Max Rate (mS)"=144, "SDI"=0, "SSM"=0, "Create SDI"=FALSE, "Create SSM"=FALSE, "Create Parity"=FALSE, "Parameter Name"="ac_date_month_tens", "Start Bit"=22, "Number of Bits"=1, "Scale"="1", "Offset"="0", "Signed"=FALSE, "Unit"="", "Encoding"=enum."BNR", "Default Value"="0"}, {"Core Number"=0, "Channel Number"=8, "Channel Name"="RDC13_NWS_RX", "Channel Speed"=100, "Label Decimal"=176, "Label Name"="Label_260", "Min Rate (mS)"=96, "Max Rate (mS)"=144, "SDI"=0, "SSM"=0, "Create SDI"=FALSE, "Create SSM"=FALSE, "Create Parity"=FALSE, "Parameter Name"="ac_date_year_ones", "Start Bit"=10, "Number of Bits"=4, "Scale"="1", "Offset"="0", "Signed"=FALSE, "Unit"="", "Encoding"=enum."BNR", "Default Value"="0"}, {"Core Number"=0, "Channel Number"=8, "Channel Name"="RDC13_NWS_RX", "Channel Speed"=100, "Label Decimal"=176, "Label Name"="Label_260", "Min Rate (mS)"=96, "Max Rate (mS)"=144, "SDI"=0, "SSM"=0, "Create SDI"=FALSE, "Create SSM"=FALSE, "Create Parity"=FALSE, "Parameter Name"="ac_date_year_tens", "Start Bit"=14, "Number of Bits"=4, "Scale"="1", "Offset"="0", "Signed"=FALSE, "Unit"="", "Encoding"=enum."BNR", "Default Value"="0"}, {"Core Number"=0, "Channel Number"=8, "Channel Name"="RDC13_NWS_RX", "Channel Speed"=100, "Label Decimal"=176, "Label Name"="Label_260", "Min Rate (mS)"=96, "Max Rate (mS)"=144, "SDI"=0, "SSM"=0, "Create SDI"=FALSE, "Create SSM"=FALSE, "Create Parity"=FALSE, "Parameter Name"="sdi", "Start Bit"=8, "Number of Bits"=2, "Scale"="1", "Offset"="0", "Signed"=FALSE, "Unit"="", "Encoding"=enum."BNR", "Default Value"="0"}, {"Core Number"=0, "Channel Number"=8, "Channel Name"="RDC13_NWS_RX", "Channel Speed"=100, "Label Decimal"=202, "Label Name"="Label_312", "Min Rate (mS)"=32, "Max Rate (mS)"=48, "SDI"=0, "SSM"=0, "Create SDI"=FALSE, "Create SSM"=FALSE, "Create Parity"=FALSE, "Parameter Name"="ground_speed", "Start Bit"=10, "Number of Bits"=19, "Scale"="0.01565", "Offset"="0", "Signed"=TRUE, "Unit"="knots", "Encoding"=enum."BNR", "Default Value"="0"}, {"Core Number"=0, "Channel Number"=8, "Channel Name"="RDC13_NWS_RX", "Channel Speed"=100, "Label Decimal"=202, "Label Name"="Label_312", "Min Rate (mS)"=32, "Max Rate (mS)"=48, "SDI"=0, "SSM"=0, "Create SDI"=FALSE, "Create SSM"=FALSE, "Create Parity"=FALSE, "Parameter Name"="sdi", "Start Bit"=8, "Number of Bits"=2, "Scale"="1", "Offset"="0", "Signed"=FALSE, "Unit"="", "Encoding"=enum."BNR", "Default Value"="0"}]) -> (8 "Active Core Numbers":i32[](array[numeric]))   [LabVIEW 2017]
uses:
  Controls/Database_Array.ctl
  Controls/Encoding.ctl
  <userlib>/_OpenG.lib/array/array.llb/Remove Duplicates from 1D Array (I32)__ogtk.vi
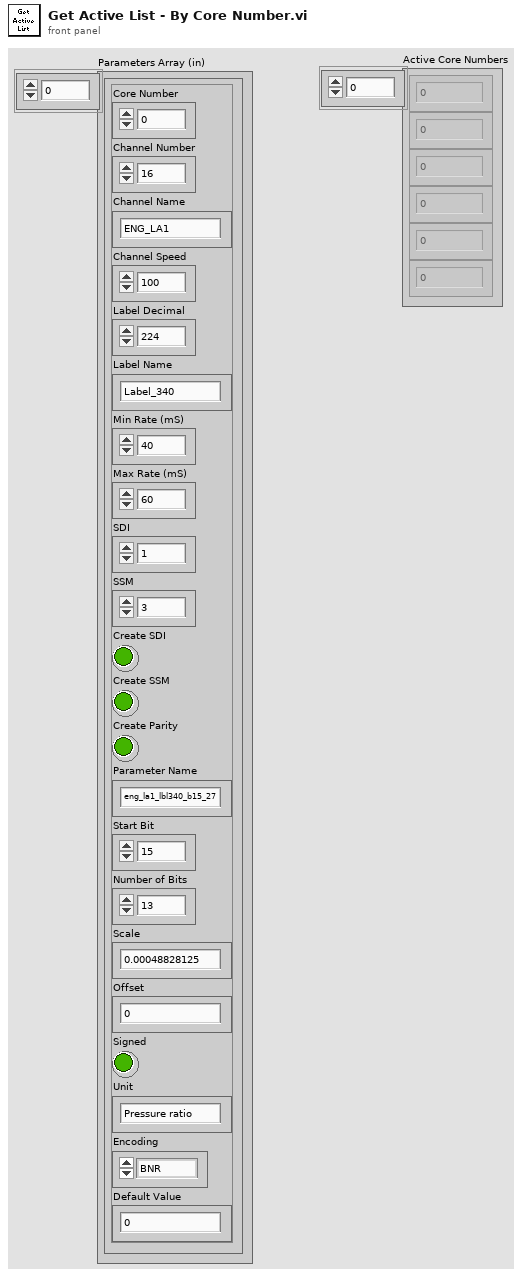
[diagram p1: front panel]
types:
  T1 = typedef "Database_Array.ctl" = cluster{"Core Number":i32, "Channel Number":i32, "Channel Name":string, "Channel Speed":i32, "Label Decimal":i32, "Label Name":string, "Min Rate (mS)":i32, "Max Rate (mS)":i32, "SDI":i32, "SSM":i32, "Create SDI":bool, "Create SSM":bool, "Create Parity":bool, "Parameter Name":string, "Start Bit":i32, "Number of Bits":i32, "Scale":string, "Offset":string, "Signed":bool, "Unit":string, "Encoding":T2, "Default Value":string}
  T2 = typedef "Encoding.ctl" = enum16{"BCD", "BNR", "Discrete"}
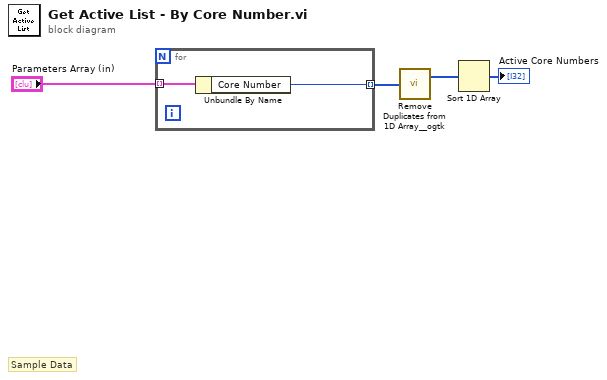
[diagram p0: block diagram]
diagram:
  # "Sample Data"
  n1 = for {
    tunnel: "Parameters Array (in)" -> [w6] mode=indexing
    tunnel: [w5] -> w3 mode=indexing
    n2 = Unbundle By Name(w6) -> ("Core Number"=w5:i32)
  }
  n3 = call-poly <userlib>:"Remove Duplicates from 1D Array__ogtk.vi"("Input Array"=w3) -> ("Output Array"=w2:i32[])  [unwired: 1 out]
  n4 = Sort 1D Array(array=w2) -> (sorted array=→"Active Core Numbers":i32[])
